vi "Update.vi"(8 "error in (no error)":errorcluster, 9 "Quem joga":string, 10 "Tabuleiro":T1, 11 "Remote in":refnum<class "Remote.lvclass">) -> (0 "error out":errorcluster, 3 "Remote out":refnum<class "Remote.lvclass">)   [LabVIEW 2019, in "Remote.lvclass"]
uses:
  Remote.lvclass
  controls/Tabuleiro.ctl
  Remote.lvclass/Remote.ctl
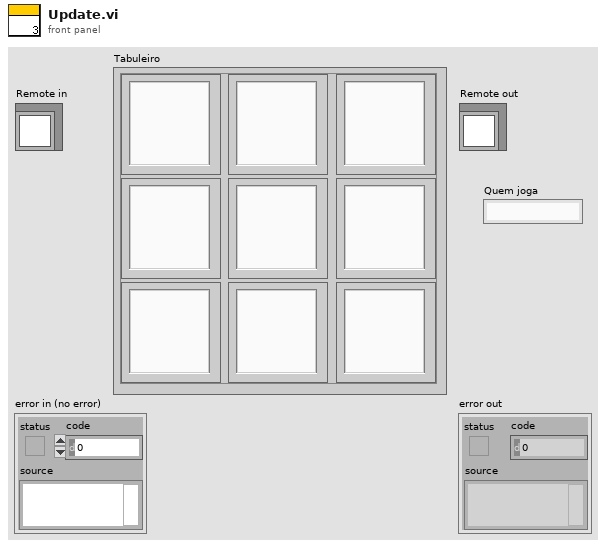
[diagram p1: front panel]
types:
  T1 = typedef "Tabuleiro.ctl" = cluster{"(0,0)":string, "(1,0)":string, "(0,1)":string, "(1,1)":string, "(2,0)":string, "(1,2)":string, "(2,2)":string, "(0,2)":string, "(2,1) ":string}
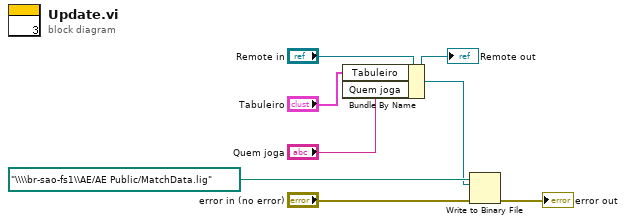
[diagram p0: block diagram]
diagram:
  n1 = Bundle By Name(cluster="Remote in", "Tabuleiro"="Tabuleiro", "Quem joga"="Quem joga") -> (w1:refnum<class "Remote.lvclass">)
  "Remote out" <- w1
  n2 = Write to Binary File(file (use dialog)=path "\\\\br-sao-fs1\\AE/AE Public/MatchData.lig", data=w1, error in="error in (no error)") -> (error out=→"error out":errorcluster)  [unwired: 3 in, 2 out]
